vi "HW_6p1_Task2_doanbs.vi"() -> ()   [LabVIEW 2016]
panel:
  out "Average Gauge Pressure":dbl
  out "Too High":dbl
  out "Too Low":dbl
  out "Acceptable Range":dbl
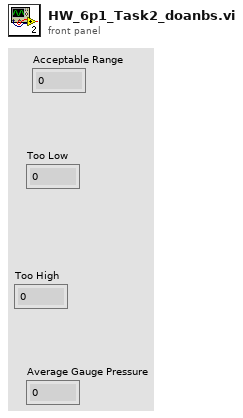
[diagram p1: front panel]
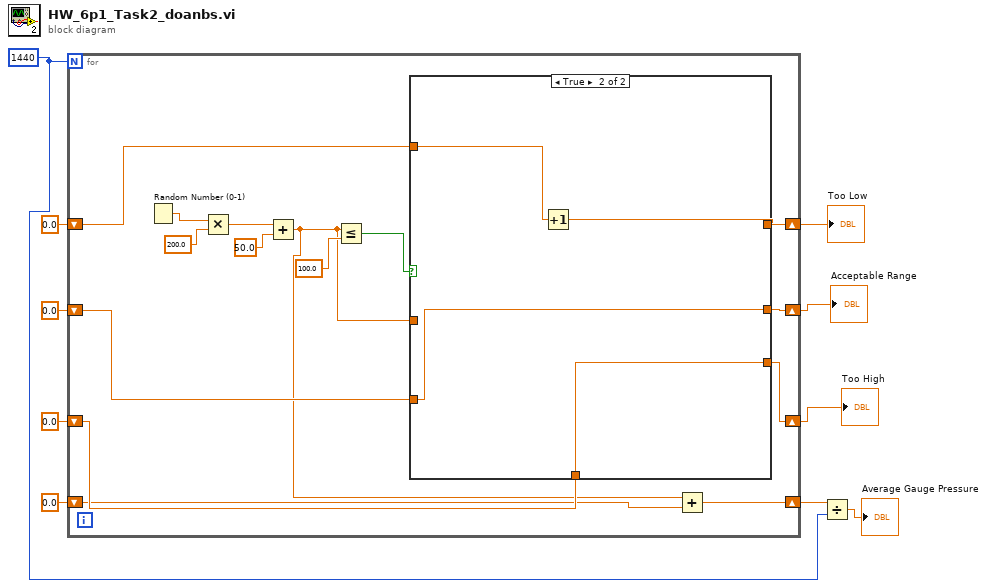
[diagram p0: block diagram]
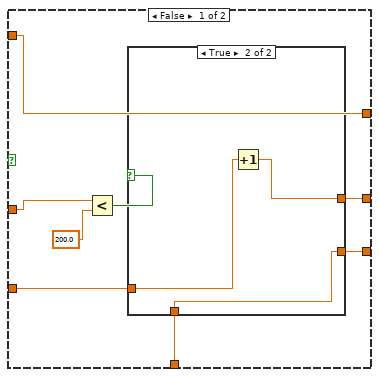
[diagram p2: hidden frame]
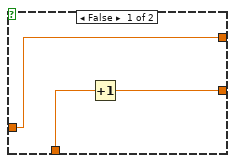
[diagram p3: hidden frame]
diagram:
  w1 = 1440
  n1 = for {
    N: w1 -> [_]
    shift-right: [w19] -> w10
    shift-left: 0.0 -> [w18]
    shift-right: [w17] -> w2
    shift-left: 0.0 -> [w16]
    shift-right: [w15] -> w9
    shift-left: 0.0 -> [w14]
    shift-right: [w13] -> w8
    shift-left: 0.0 -> [w11]
    n2 = Random Number (0-1)() -> (number: 0 to 1=w24:dbl)
    n3 = Multiply(x=w24, y=200.0) -> (x*y=w23:dbl)
    n4 = Add(x=w23, y=50.0) -> (x+y=w12:dbl)
    n5 = Less Or Equal?(x=w12, y=100.0) -> (x <= y?=w20:bool)
    n6 = case shown="True" w20 {
      tunnel: [w33 w43] -> w19
      tunnel: w18 -> [w33 w42]
      tunnel: w12 -> [w31 _]
      tunnel: [w29 w41] -> w17
      tunnel: w16 -> [w28 w41]
      tunnel: [w27 w40] -> w15
      tunnel: w14 -> [w26 w40]
      frame False {
        n7 = Less?(x=w31, y=200.0) -> (x < y?=w30:bool)
        n8 = case shown="True" w30 {
          tunnel: [w34 w39] -> w29
          tunnel: w28 -> [w34 w38]
          tunnel: [w36 w37] -> w27
          tunnel: w26 -> [w35 w37]
          frame False {
            n9 = Increment(x=w35) -> (x+1=w36:dbl)
          }
          frame True {
            n10 = Increment(x=w38) -> (x+1=w39:dbl)
          }
        }
      }
      frame True {
        n11 = Increment(x=w42) -> (x+1=w43:dbl)
      }
    }
    n12 = Add(x=w12, y=w11) -> (x+y=w13:dbl)
  }
  "Too Low" <- w10
  "Too High" <- w9
  "Acceptable Range" <- w2
  n13 = Divide(x=w8, y=w1) -> (x/y=→"Average Gauge Pressure":dbl)
